vi "PID (SGL).vi"(0 "process variable":sgl, 1 "reset":bool, 7 "setpoint":sgl, 12 "PID gains":T1, 13 "output range":cluster{"output high":sgl, "output low":sgl}={"output high"=32767.0, "output low"=-32768.0}) -> (4 "output":sgl)   [LabVIEW 2014]
doc: "On an FPGA target, implements an integer PID algorithm for PID applications with high-speed control and/or high channel count that require an efficient algorithm. You can use this Express VI with single-channel or multi-channel configurations. The PID algorithm features control action range and uses the integrator anti-windup calculation to limit the effect of the integral action during transients. The PID algorithm also features bumpless controller output for PID gain changes.\n--------------------\n\nThis Express VI is configured as follows:\n\nNumber of channels = 1\nProportional gain (Kc) = 1\nIntegral time (Ti) = 9.99219mmin\nDerivative time (Td) = 0min\nSampling time (Ts) = 1s\nProportional gain (scaled) (Kc * 2^8) = 256\nIntegral gain (scaled) ([Kc*Ts]/[Ti*60] * 2^8) = 427\nDerivative gain (scaled) ([Kc*Td*60]/[Ts] * 2^8) = 0\nOutput range high = 0\nOutput range low = 0\nInitial setpoint = 0"
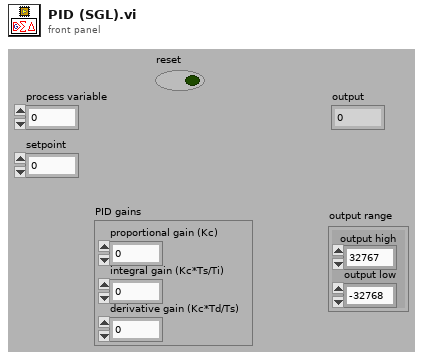
[diagram p1: front panel]
types:
  T1 = cluster{"proportional gain (Kc)":sgl, "integral gain (Kc*Ts/Ti)":sgl, "derivative gain (Kc*Td/Ts)":sgl}
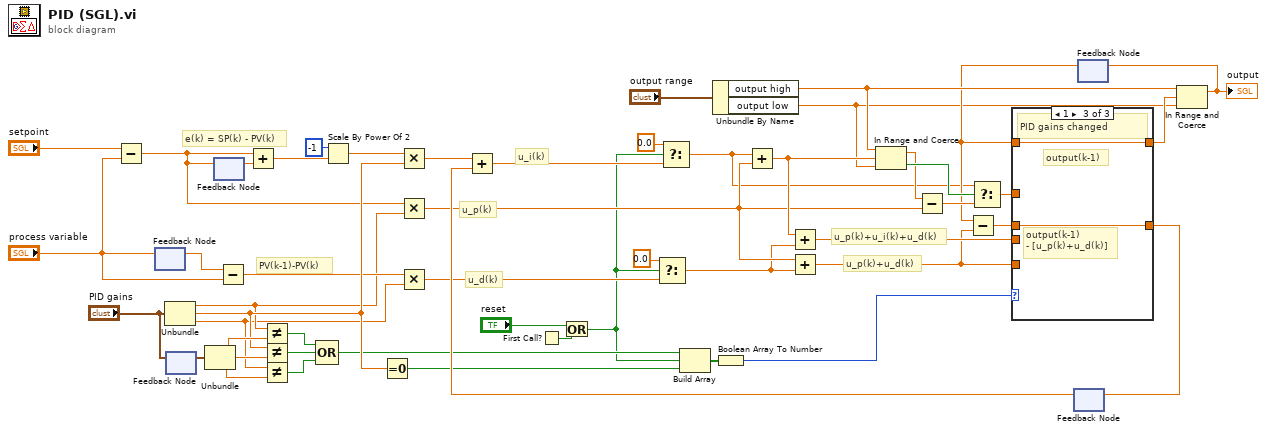
[diagram p0: block diagram]
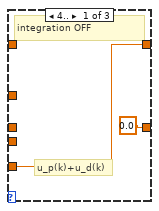
[diagram p2: hidden frame]
diagram:
  # "u_i(k)"
  # "u_p(k)"
  # "u_p(k)+u_i(k)+u_d(k)"
  # "u_p(k)+u_d(k)"
  # "u_d(k)"
  # "PV(k-1)-PV(k)"
  # "e(k) = SP(k) - PV(k)"
  n1 = Subtract(x="setpoint", y="process variable") -> (x-y=w27:sgl)
  n2 = feedback #1() -> (w32:sgl)  [unwired: 1 in]
  n3 = feedback-in #1("process variable") -> ()
  n4 = Unbundle("PID gains") -> ("proportional gain (Kc)"=w30:sgl, "integral gain (Kc*Ts/Ti)"=w37:sgl, "derivative gain (Kc*Td/Ts)"=w29:sgl)
  n5 = feedback #2() -> (w46:T1)  [unwired: 1 in]
  n6 = feedback-in #2("PID gains") -> ()
  n7 = Unbundle(w46) -> ("proportional gain (Kc)"=w45:sgl, "integral gain (Kc*Ts/Ti)"=w43:sgl, "derivative gain (Kc*Td/Ts)"=w41:sgl)
  n8 = feedback #3() -> (w31:sgl)  [unwired: 1 in]
  n9 = feedback-in #3(w27) -> ()
  n10 = Subtract(x=w32, y="process variable") -> (x-y=w33:sgl)
  n11 = Add(x=w27, y=w31) -> (x+y=w34:sgl)
  n12 = Not Equal?(x=w30, y=w45) -> (x != y?=w44:bool)
  n13 = Not Equal?(x=w37, y=w43) -> (x != y?=w42:bool)
  n14 = Not Equal?(x=w29, y=w41) -> (x != y?=w40:bool)
  n15 = Compound Arithmetic op=OR(w44, w42, w40) -> (w9:bool)
  n16 = Scale By Power Of 2(n=i8 -1, x=w34) -> (x*2^n=w28:sgl)
  n17 = Equal To 0?(x=w37) -> (x = 0?=w13:bool)
  n18 = Multiply(x=w28, y=w37) -> (x*y=w36:sgl)
  n19 = Multiply(x=w27, y=w30) -> (x*y=w12:sgl)
  n20 = Multiply(x=w33, y=w29) -> (x*y=w3:sgl)
  n21 = First Call?() -> (First Call?: T/F=w39:bool)
  n22 = Or(x="reset", y=w39) -> (x .or. y?=w2:bool)
  n23 = Select(t=sgl 0.0, s=w2, f=w3) -> (s? t:f=w1:sgl)
  n24 = Build Array(w9, w2, w13) -> (w22:bool[])
  n25 = Unbundle By Name("output range") -> ("output high"=w15:sgl, "output low"=w8:sgl)
  n26 = Boolean Array To Number(Boolean array=w22) -> (number=w21:u8)
  n27 = Add(x=w12, y=w1) -> (x+y=w16:sgl)
  n28 = feedback #4() -> (w38:sgl)  [unwired: 1 in]
  n29 = Add(x=w36, y=w38) -> (x+y=w6:sgl)
  n30 = Select(t=sgl 0.0, s=w2, f=w6) -> (s? t:f=w5:sgl)
  n31 = Add(x=w5, y=w12) -> (x+y=w23:sgl)
  n32 = Add(x=w23, y=w1) -> (x+y=w18:sgl)
  n33 = In Range and Coerce(upper limit=w15, x=w23, lower limit=w8) -> (coerced(x)=w25:sgl, In Range?=w26:bool)
  n34 = Subtract(x=w25, y=w12) -> (x-y=w24:sgl)
  n35 = Select(t=w5, s=w26, f=w24) -> (s? t:f=w19:sgl)
  n36 = feedback #5() -> (w14:sgl)  [unwired: 1 in]
  n37 = Subtract(x=w14, y=w16) -> (x-y=w17:sgl)
  n38 = case shown="1" w21 {
    tunnel: [sgl 0.0 ("t") w55 w57] -> w11
    tunnel: [w53 w54 w56] -> w20
    tunnel: w16 -> [w53 _ _]
    tunnel: w17 -> [_ _ w57]
    tunnel: w18 -> [_ w54 _]
    tunnel: w19 -> [_ w55 _]
    tunnel: w14 -> [_ _ w56]
    frame 4.. {
      # "u_p(k)+u_d(k)"
      # "integration OFF"
    }
    frame Default {
      # "normal PID"
    }
    frame 1 {
      # "output(k-1)"
      # "output(k-1)\n- [u_p(k)+u_d(k)]"
      # "PID gains changed"
    }
  }
  n39 = feedback-in #4(w11) -> ()
  n40 = In Range and Coerce(upper limit=w15, x=w20, lower limit=w8) -> (coerced(x)=w10:sgl)  [unwired: 1 out]
  "output" <- w10
  n41 = feedback-in #5(w10) -> ()
